vi "Send Command.vi"(7 "Timeout (100 ms)":i32=100, 8 "Error In":errorcluster, 9 "ARGS":u8[](array[numeric]), 10 "CMD":u16, 11 "LINX Device Config":T1) -> (0 "Error Out":errorcluster, 1 "Status":u8, 2 "Response":u8[](array[numeric]), 3 "LINX Device Config":T1)   [LabVIEW 2014, in "LMH-LINX.lvlib" / "Device.lvlib"]
doc: "Send a packet to the LINX device and return the LINX device response packet."
uses:
  Device.lvlib
  Type Defs/LINX Device Config.ctl
  Type Defs/Interface.ctl
  Type Defs/TCP Config.ctl
  Type Defs/Channels.ctl
  Type Defs/Error Type.ctl
  LMH-LINX.lvlib
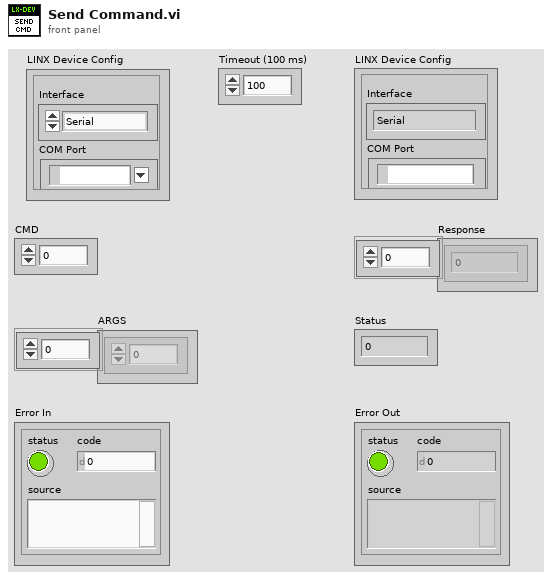
[diagram p1: front panel]
types:
  T1 = typedef "LMH-LINX.lvlib/Device.lvlib/LINX Device Config.ctl" = cluster{"Interface":T2, "COM Port":refnum<visa-resource-name>, "TCP Configuration":T3, "Device Family":u8, "Device ID":u8, "Device Name":string, "TCP Ref":refnum<k5>, "Channels":T4}
  T2 = typedef "LMH-LINX.lvlib/Interface.ctl" = enum16{"Serial", "TCP"}
  T3 = typedef "LMH-LINX.lvlib/Device.lvlib/TCP Config.ctl" = cluster{"IP Address":string, "Port":u16}
  T4 = typedef "LMH-LINX.lvlib/Channels.ctl" = cluster{"DI":u8[], "DO":u8[], "AI":u8[], "AO":u8[], "PWM":u8[], "QE":u8[], "UART":u8[], "I2C 2":u8[], "SPI":u8[], "CAN":u8[], "Servo":u8[], "AI Ref (V)":dbl, "AO Ref (V)":dbl, "AO Resolution (Bits)":u8}
  T5 = typedef "LMH-LINX.lvlib/Error Type.ctl" = enum16{"Unknown", "Timeout", "Corrupt Return Packet", "Unable To Connect", "Command Not Supported", "Channel DNE", "Invalid COM Config", "Firmware Version Mismatch", "myRIO Support", "CMD Specific Error"}
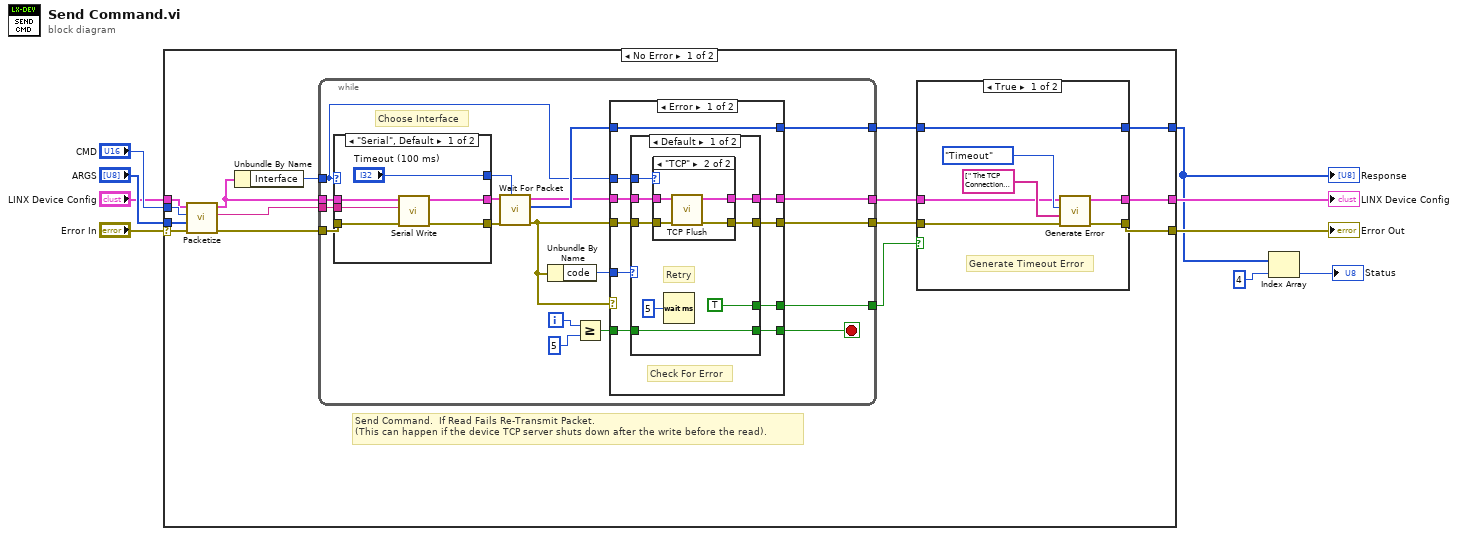
[diagram p0: block diagram]
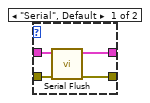
[diagram p3: hidden frame]
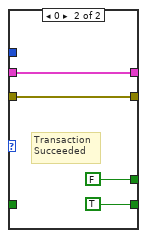
[diagram p4: hidden frame]
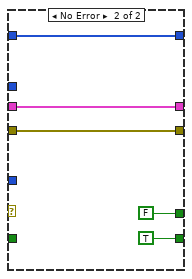
[diagram p5: hidden frame]
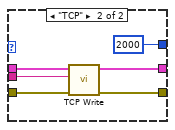
[diagram p6: hidden frame]
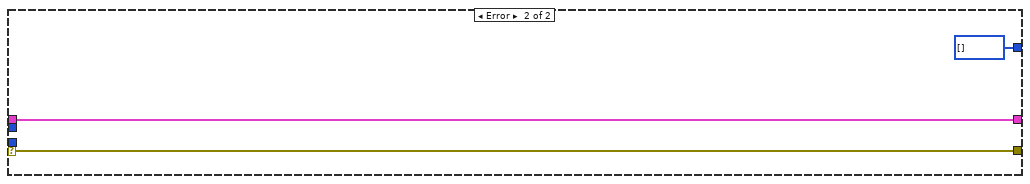
[diagram p7: hidden frame]
diagram:
  n1 = case shown="No Error" "Error In" {
    selector: "Error In" -> [w11 w101]
    tunnel: "ARGS" -> [w22 _]
    tunnel: "CMD" -> [w21 _]
    tunnel: "LINX Device Config" -> [w18 w103]
    tunnel: [w17 w103] -> w6
    tunnel: [w16 w101] -> w5
    tunnel: [w13 u8[] [] ("Packet")] -> w3
    frame No Error {
      # "Send Command.  If Read Fails Re-Transmit Packet.\n(This can happen if the device TCP server shuts down after the write before the read)."
      n2 = call "Packetize.vi"("Error In"=w11, "ARGS"=w22, "CMD"=w21, "LINX Device Config"=w18) -> ("Error Out"=w24:errorcluster, "Packet"=w23:string, "LINX Decice Config"=w20:T1)  [unwired: 5 in]
      n3 = Unbundle By Name(w20) -> ("Interface"=w19:T2)
      n4 = while {
        tunnel: w24 -> [w53]
        tunnel: w23 -> [w52]
        tunnel: w20 -> [w51]
        tunnel: w19 -> [w35]
        tunnel: [w40] -> w12
        tunnel: [w44] -> w15
        tunnel: [w37] -> w14
        tunnel: [w41] -> w10
        i -> [w48]
        stop <- w43 stop-if-true
        # "Choose Interface"
        n5 = case shown="\"Serial\", Default" w35 {
          tunnel: w51 -> [w93 w98]
          tunnel: w53 -> [w94 w99]
          tunnel: [w90 w96] -> w50
          tunnel: [w91 w97] -> w49
          tunnel: w52 -> [w92 w100]
          tunnel: ["Timeout (100 ms)" 2000 ("Timeout (100 ms)")] -> w46
          frame "Serial", Default {
            n6 = call "Serial Write.vi"("Error In"=w94, "Data"=w92, "LINX Device Config"=w93) -> ("Error Out"=w90:errorcluster, "LINX Device Config"=w91:T1)  [unwired: 7 in]
          }
          frame "TCP" {
            n7 = call "TCP Write.vi"("Error In"=w99, "Packet"=w100, "LINX Decice Config"=w98) -> ("Error Out"=w96:errorcluster, "LINX Decice Config"=w97:T1)  [unwired: 7 in]
          }
        }
        n8 = call "Wait For Packet.vi"("Timeout (100 ms)"=w46, "Error In"=w50, "LINX Device Config"=w49) -> ("Error Out"=w36:errorcluster, "Packet"=w39:u8[], "LINX Device Config"=w38:T1)  [unwired: 6 in]
        n9 = Unbundle By Name(w36) -> ("code"=w45:i32)
        n10 = Greater Or Equal?(x=w48, y=5) -> (x >= y?=w42:bool)
        n11 = case shown="Error" w36 {
          tunnel: w45 -> [w63 _]
          tunnel: [w62 w88] -> w44
          tunnel: [w61 TRUE] -> w43
          tunnel: w42 -> [w60 _]
          tunnel: [w59 FALSE] -> w41
          tunnel: [w58 w84] -> w40
          tunnel: w39 -> [w58 w84]
          tunnel: w38 -> [w57 w85]
          tunnel: [w56 w85] -> w37
          tunnel: w36 -> [w55 w88]
          tunnel: w35 -> [w54 _]
          frame Error {
            # "Check For Error"
            n12 = case shown="Default" w63 {
              tunnel: [w66 w83] -> w62
              tunnel: [w71 TRUE] -> w61
              tunnel: w60 -> [w71 _]
              tunnel: [TRUE FALSE] -> w59
              tunnel: w57 -> [w68 w80]
              tunnel: [w67 w80] -> w56
              tunnel: w55 -> [w65 w83]
              tunnel: w54 -> [w64 _]
              frame Default {
                # "Retry"
                n13 = case shown="\"TCP\"" w64 {
                  tunnel: w68 -> [w75 w79]
                  tunnel: [w74 w78] -> w67
                  tunnel: [w73 w77] -> w66
                  tunnel: w65 -> [w72 w76]
                  frame "Serial", Default {
                    n14 = call "Serial Flush.vi"("Error In"=w72, "LINX Device Config"=w75) -> ("Error Out"=w73:errorcluster, "LINX Device Config"=w74:T1)  [unwired: 8 in]
                  }
                  frame "TCP" {
                    n15 = call "TCP Flush.vi"("Error In"=w76, "LINX Device Config"=w79) -> ("Error Out"=w77:errorcluster, "LINX Device Config"=w78:T1)  [unwired: 7 in, 1 out]
                  }
                }
                n16 = Wait (ms)(milliseconds to wait=u32 5) -> ()  [unwired: 1 out]
              }
              frame 0 {
                # "Transaction \nSucceeded"
              }
            }
          }
          frame No Error {
          }
        }
      }
      n17 = case shown="True" w10 {
        tunnel: [w31 w32] -> w16
        tunnel: [w28 w33] -> w17
        tunnel: w15 -> [w27 w32]
        tunnel: w14 -> [w26 w33]
        tunnel: [w25 w34] -> w13
        tunnel: w12 -> [w25 w34]
        frame True {
          # "Generate Timeout Error"
          n18 = call "Generate Error.vi"("Error In"=w27, "Arguments"=string[] [" The TCP Connection Was Refused."], "Error Type"=Error_Type."Timeout", "LINX Device Config"=w26) -> ("Error Out"=w31:errorcluster, "LINX Device Config"=w28:T1)  [unwired: 6 in]
        }
        frame False {
          # "Send/Rec Successful\nNo Error"
        }
      }
    }
    frame Error {
    }
  }
  "Error Out" <- w5
  "Response" <- w3
  "LINX Device Config" <- w6
  n19 = Index Array(array=w3, index=4 ("x")) -> (element=→"Status":u8)
